vi "Process.vi"(8 "error in (no error)":errorcluster, 11 "Report Generator In":refnum<class "Report Generator.lvclass">) -> (0 "error out":errorcluster, 3 "Report Generator Out":refnum<class "Report Generator.lvclass">)   [LabVIEW 2020, in "Report Generator.lvclass"]
uses:
  Report Generator.lvclass
  C:/Git/astemes-lunit/source/Application Framework/Process Classes/Process/Process.lvclass
  Report Generator.lvclass/Report Generator.ctl
  Report Classes/XML Report/XML Report.lvclass
  Result Collector/Result Collector.lvclass/Result Collector.ctl
  Result Types/Suite Results/Test Suite Result.ctl
  Result Types/Case Result/Test Case Result.ctl
  Result Types/Method Result/Method Result.ctl
  Rewrite Project/Result/Status.ctl
  Result Types/Assertion Result/Assertion Result.ctl
  Result Types/Assertion Result/Public/TypeDefs/Assertion Type.ctl
  Application Framework/Process Classes/Process/Process.lvclass/Process.ctl
  Result Collector/Result Collector.lvclass
  Report Classes/Test Report/Test Report.lvclass/Test Report.ctl
  Report Classes/Test Report/Test Report.lvclass
  Result Types/Suite Results/Public/Read Errors count.vi
  Result Types/Suite Results/Public/Read Test Method Count.vi
  Result Types/Suite Results/Public/Read Test Case count.vi
  Result Types/Suite Results/Public/Read Failed count.vi
  Result Types/Suite Results/Public/Read Execution time.vi
  Result Types/Suite Results/Public/Read Passed count.vi
  Result Types/Suite Results/Public/Read Skipped count.vi
  Application Framework/Process Classes/Process/Public/Accessors/Read Process Name.vi
  Result Types/Suite Results/Private/Count by Status.vi
  Result Types/Case Result/Public/Read Test Method Count.vi
  Result Types/Case Result/Public/Read Status.vi
  Result Types/Case Result/Private/Merge Status.vi
  Result Types/Method Result/Public/Read Status.vi
  <vilib>/Utility/error.llb/Error Cluster From Error Code.vi
  Application Framework/Process Classes/Error Handler/Private/SubVIs/Get Error Queue Name.vi
  Application Framework/Process Classes/Process/Process.lvclass
  Application Framework/Process Classes/Error Handler/Error Handler.lvclass
  Result Types/Case Result/Test Case Result.lvlib
  Result Types/Suite Results/Test Suite Result.lvlib
  Rewrite Project/Result/Result.lvlib
  Result Types/Assertion Result/Assertion Result.lvlib
  Result Types/Method Result/Method Result.lvlib
panel:
  out "Stopped":bool
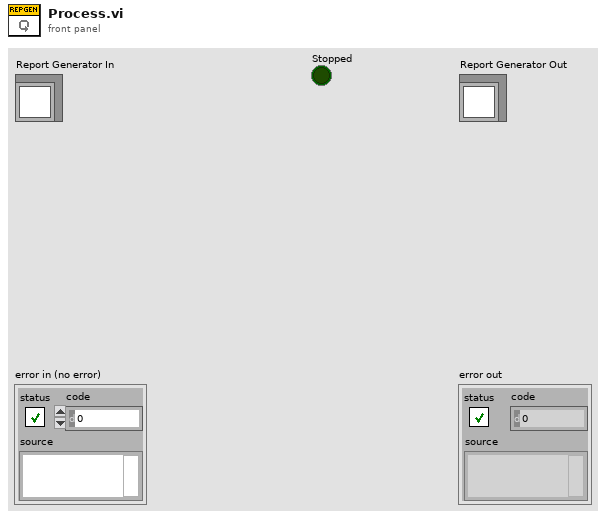
[diagram p1: front panel]
types:
  T1 = typedef "Test Suite Result.lvlib/Test Suite Result.ctl" = cluster{"Test Suite ID":string, "Name":string, "Hostname":string, "Status":T2, "Execution time":dbl, "Start Time":timestamp, "Case Results":T3[]}
  T2 = typedef "Result.lvlib/Status.ctl" = enum16{"Pass", "Fail", "Error", "Skipped", "Setup Error", "Broken", "Teardown Error"}
  T3 = typedef "Test Case Result.lvlib/Test Case Result.ctl" = map{string, T4}
  T4 = typedef "Method Result.lvlib/Method Result.ctl" = cluster{"Test Case":string, "Test Method Name":string, "Status":T2, "Assertion Results":T5[], "Execution time":dbl, "Result String":string}
  T5 = typedef "Assertion Result.lvlib/Assertion Result.ctl" = cluster{"Status":T2, "Message":string, "Description":string, "Assertion Type":T6}
  T6 = typedef "Result.lvlib/Assertion Type.ctl" = enum16{"None", "Pass", "Fail", "Skip", "Pass if Equal", "Fail if Equal", "Pass if Error", "Fail if Error", "Pass if", "Fail if"}
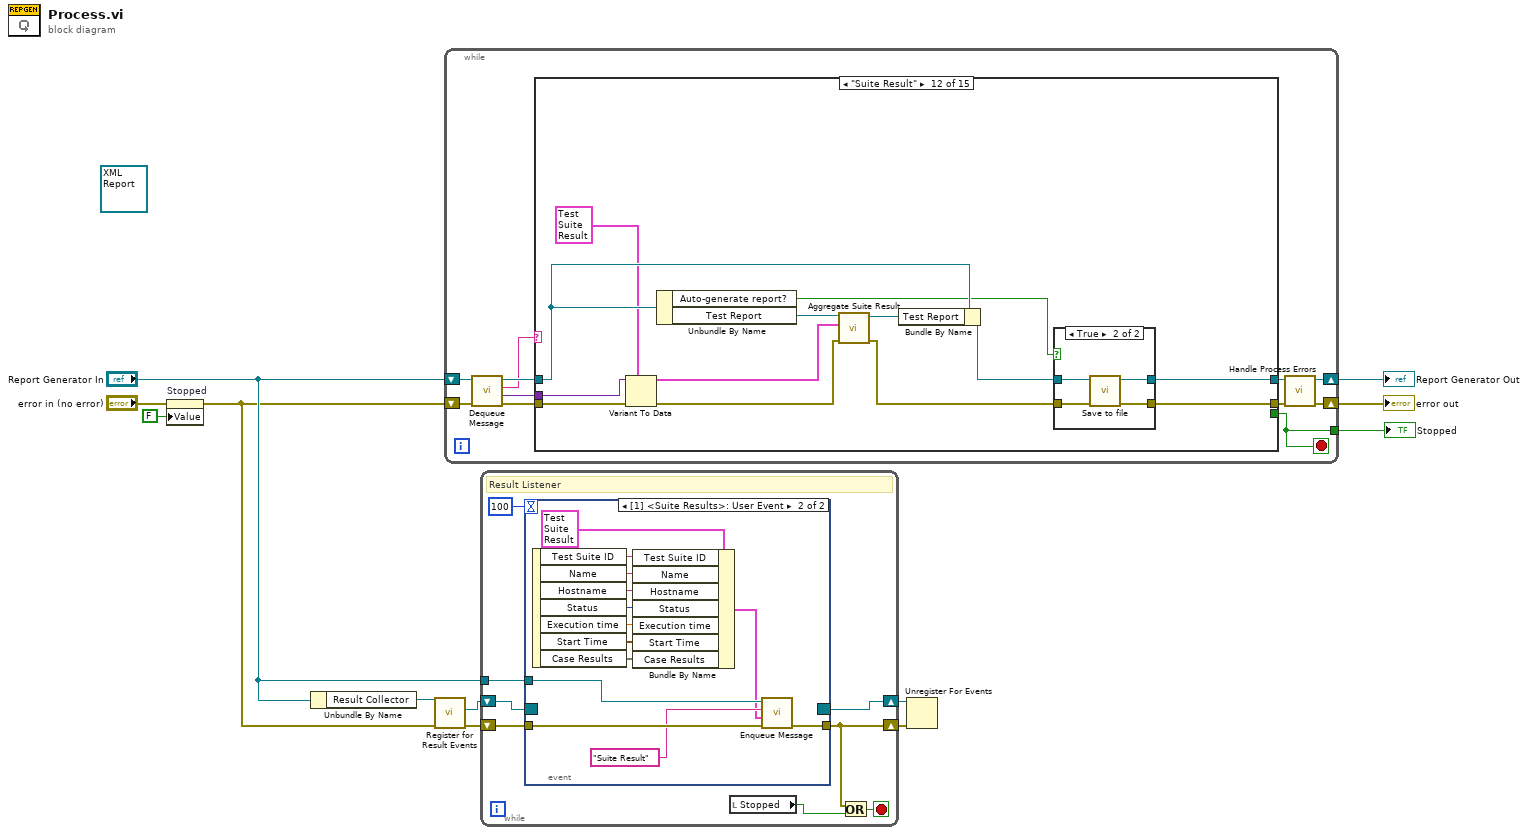
[diagram p0: block diagram]
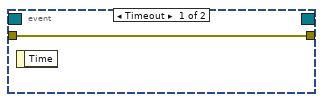
[diagram p2: hidden frame]
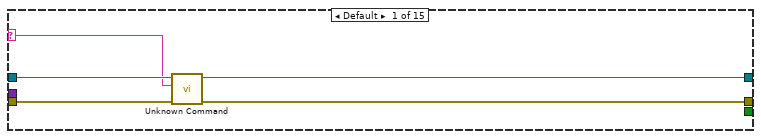
[diagram p3: hidden frame]
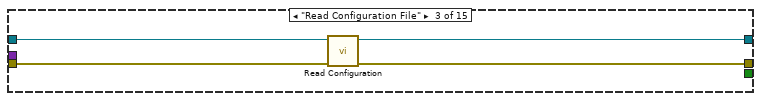
[diagram p5: hidden frame]
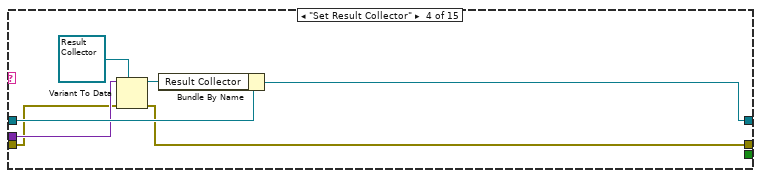
[diagram p6: hidden frame]
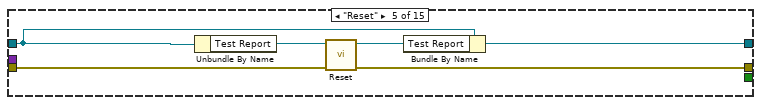
[diagram p7: hidden frame]
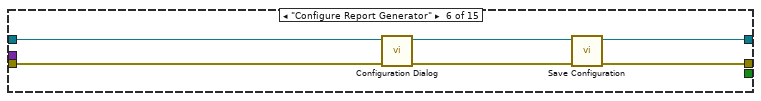
[diagram p8: hidden frame]
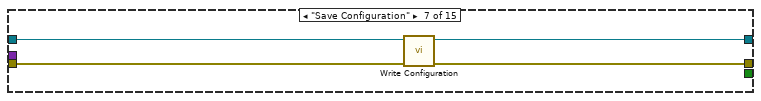
[diagram p9: hidden frame]
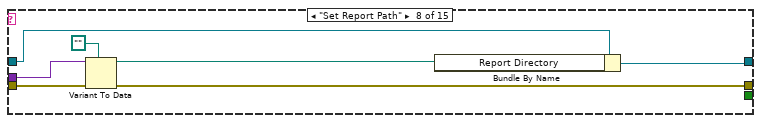
[diagram p10: hidden frame]
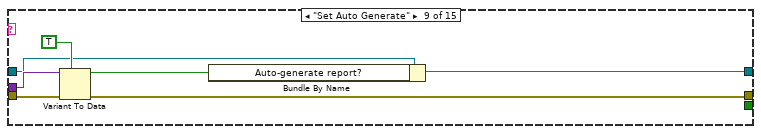
[diagram p11: hidden frame]
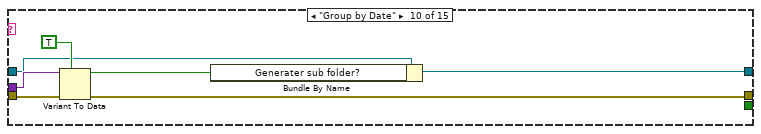
[diagram p12: hidden frame]
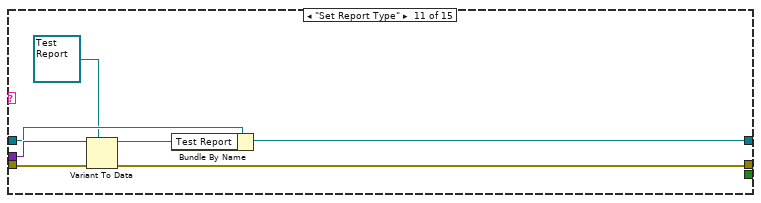
[diagram p13: hidden frame]
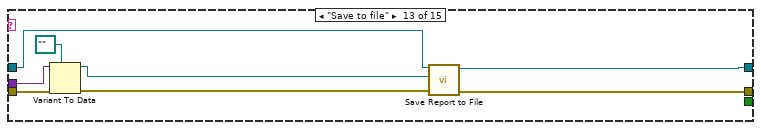
[diagram p15: hidden frame]
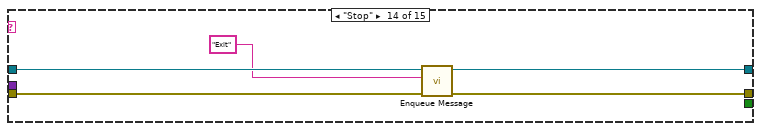
[diagram p16: hidden frame]
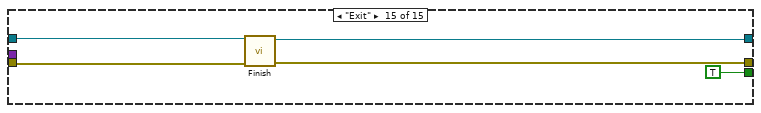
[diagram p17: hidden frame]
diagram:
  (unwired) refnum<class "XML Report.lvclass"> refnum ("XML Report.lvclass")
  n1 = property on="Stopped" class="Bool (strict)"(error in="error in (no error)", "Value"=FALSE ("Stopped")) -> (error out=w1:errorcluster)  [unwired: 1 in, 1 out]
  n2 = Unbundle By Name("Report Generator In") -> ("Result Collector"=w10:refnum<class "Result Collector.lvclass">)
  n3 = call "Register for Result Events.vi"("error in (no error)"=w1, "Result Collector In"=w10) -> ("error out"=w8:errorcluster, "Event Registration Refnum"=w9:refnum<event-registration>)  [unwired: 7 in, 1 out]
  n4 = while {
    shift-right: [w16] -> w12
    shift-left: w1 -> [w22]
    shift-right: [w17] -> w11
    shift-left: "Report Generator In" -> [w23]
    tunnel: [w13] -> w4
    stop <- w13 stop-if-true
    n5 = call "Dequeue Message.vi"("error in (no error)"=w22, "Process In"=w23) -> ("error out"=w21:errorcluster, "Message Data"=w14:variant, "Message"=w18:string, "Process Out"=w19:refnum<class "Report Generator.lvclass">)  [unwired: 6 in]
    n6 = case shown="\"Suite Result\"" w18 {
      selector: w18 -> [w24 _ _ _ _ _ _ _ _ _ _ _ _ _ _]
      tunnel: [w26 w29 w31 w35 w43 w49 w54 w58 w66 w73 w81 w88 w107 w114 w119] -> w15
      tunnel: w21 -> [w25 w29 w32 w39 w44 w52 w55 w64 w71 w78 w85 w96 w112 w116 w121]
      tunnel: [w28 w30 w33 w36 w42 w48 w56 w60 w65 w72 w80 w90 w106 w115 w120] -> w20
      tunnel: w19 -> [w27 w30 w34 w41 w45 w53 w57 w61 w68 w75 w83 w98 w109 w117 w122]
      tunnel: [_ _ _ _ _ _ _ _ _ _ _ _ _ _ TRUE] -> w13
      tunnel: w14 -> [_ _ _ w40 _ _ _ w63 w70 w77 w84 w93 w111 _ _]
      frame Default {
        n7 = call "Unknown Command.vi"("error in (no error)"=w25, "String"=w24, "Process In"=w27) -> ("error out"=w26:errorcluster, "Process Out"=w28:refnum<class "Report Generator.lvclass">)  [unwired: 7 in]
      }
      frame "Init" {
      }
      frame "Read Configuration File" {
        n8 = call-dynamic "Read Configuration.vi"("error in (no error)"=w32, "Report Generator In"=w34) -> ("error out"=w31:errorcluster, "Report Generator Out"=w33:refnum<class "Report Generator.lvclass">)  [unwired: 8 in]
      }
      frame "Set Result Collector" {
        n9 = Variant To Data(error in=w39, type=refnum<class "Result Collector.lvclass"> refnum ("Result Collector"), Variant=w40) -> (data=w37:refnum<class "Result Collector.lvclass">, error out=w35:errorcluster)
        n10 = Bundle By Name(cluster=w41, "Result Collector"=w37) -> (w36:refnum<class "Report Generator.lvclass">)
      }
      frame "Reset" {
        n11 = Unbundle By Name(w45) -> ("Test Report"=w47:refnum<class "Test Report.lvclass">)
        n12 = call "Reset.vi"("error in (no error)"=w44, "Report In"=w47) -> ("error out"=w43:errorcluster, "Report Out"=w46:refnum<class "Test Report.lvclass">)  [unwired: 8 in]
        n13 = Bundle By Name(cluster=w45, "Test Report"=w46) -> (w42:refnum<class "Report Generator.lvclass">)
      }
      frame "Configure Report Generator" {
        n14 = call "Configuration Dialog.vi"("error in (no error)"=w52, "Report Generator In"=w53) -> ("error out"=w50:errorcluster, "Report Generator Out"=w51:refnum<class "Report Generator.lvclass">)  [unwired: 8 in]
        n15 = call "Save Configuration.vi"("error in (no error)"=w50, "Report Generator in"=w51) -> ("error out"=w49:errorcluster, "Report Generator out"=w48:refnum<class "Report Generator.lvclass">)  [unwired: 8 in]
      }
      frame "Save Configuration" {
        n16 = call-dynamic "Write Configuration.vi"("error in (no error)"=w55, "Report Generator In"=w57) -> ("error out"=w54:errorcluster, "Report Generator Out"=w56:refnum<class "Report Generator.lvclass">)  [unwired: 8 in]
      }
      frame "Set Report Path" {
        n17 = Variant To Data(error in=w64, type=path "", Variant=w63) -> (data=w59:path, error out=w58:errorcluster)
        n18 = Bundle By Name(cluster=w61, "Report Directory"=w59) -> (w60:refnum<class "Report Generator.lvclass">)
      }
      frame "Set Auto Generate" {
        n19 = Variant To Data(error in=w71, type=TRUE, Variant=w70) -> (data=w67:bool, error out=w66:errorcluster)
        n20 = Bundle By Name(cluster=w68, "Auto-generate report?"=w67) -> (w65:refnum<class "Report Generator.lvclass">)
      }
      frame "Group by Date" {
        n21 = Variant To Data(error in=w78, type=TRUE, Variant=w77) -> (data=w74:bool, error out=w73:errorcluster)
        n22 = Bundle By Name(cluster=w75, "Generater sub folder?"=w74) -> (w72:refnum<class "Report Generator.lvclass">)
      }
      frame "Set Report Type" {
        n23 = Variant To Data(error in=w85, type=refnum<class "Test Report.lvclass"> refnum ("Test Report.lvclass"), Variant=w84) -> (data=w82:refnum<class "Test Report.lvclass">, error out=w81:errorcluster)
        n24 = Bundle By Name(cluster=w83, "Test Report"=w82) -> (w80:refnum<class "Report Generator.lvclass">)
      }
      frame "Suite Result" {
        n25 = Variant To Data(error in=w96, type=T1 {"Test Suite ID"="", "Name"="", "Hostname"="", "Status"=enum."Pass", "Execution time"=0.0, "Start Time"=timestamp(0 s since 1904-01-01), "Case Results"=[]} ("Cluster of class private data"), Variant=w93) -> (data=w92:T1, error out=w94:errorcluster)
        n26 = Unbundle By Name(w98) -> ("Auto-generate report?"=w87:bool, "Test Report"=w97:refnum<class "Test Report.lvclass">)
        n27 = call "Aggregate Suite Result.vi"("error in (no error)"=w94, "Test Suite Result"=w92, "Report In"=w97) -> ("error out"=w89:errorcluster, "Report Out"=w95:refnum<class "Test Report.lvclass">)  [unwired: 7 in]
        n28 = Bundle By Name(cluster=w98, "Test Report"=w95) -> (w91:refnum<class "Report Generator.lvclass">)
        n29 = case shown="True" w87 {
          tunnel: w91 -> [w100 w104]
          tunnel: [w100 w103] -> w90
          tunnel: w89 -> [w99 w102]
          tunnel: [w99 w101] -> w88
          frame False {
          }
          frame True {
            n30 = call "Save to file.vi"("error in (no error)"=w102, "Report Generator In"=w104) -> ("error out"=w101:errorcluster, "Report Generator Out"=w103:refnum<class "Report Generator.lvclass">)  [unwired: 8 in]
          }
        }
      }
      frame "Save to file" {
        n31 = Variant To Data(error in=w112, type=path "", Variant=w111) -> (data=w105:path, error out=w108:errorcluster)
        n32 = call "Save Report to File.vi"("error in (no error)"=w108, "Report Directory"=w105, "Report Generator in"=w109) -> ("error out"=w107:errorcluster, "Report Generator out"=w106:refnum<class "Report Generator.lvclass">)  [unwired: 7 in]
      }
      frame "Stop" {
        n33 = call "Enqueue Message.vi"("error in (no error)"=w116, "Message"="Exit", "Process In"=w117) -> ("error out"=w114:errorcluster, "Process Out"=w115:refnum<class "Report Generator.lvclass">)  [unwired: 7 in]
      }
      frame "Exit" {
        n34 = call "Finish.vi"("error in (no error)"=w121, "Process In"=w122) -> ("error out"=w119:errorcluster, "Process Out"=w120:refnum<class "Report Generator.lvclass">)  [unwired: 8 in]
      }
    }
    n35 = call "Handle Process Errors.vi"("error in (no error)"=w15, "Process In"=w20) -> ("error out"=w16:errorcluster, "Process Out"=w17:refnum<class "Report Generator.lvclass">)  [unwired: 8 in]
  }
  "error out" <- w12
  "Report Generator Out" <- w11
  "Stopped" <- w4
  n36 = while {
    tunnel: "Report Generator In" -> [w128]
    shift-right: [w127] -> w6
    shift-left: w9 -> [w130]
    shift-right: [w125] -> w5
    shift-left: w8 -> [w129]
    stop <- w124 stop-if-true
    # "Result Listener"
    n37 = event shown="[1] <Suite Results>: User Event" {
      selector: w130 -> [_ _]
      dyn-events: [_ _] -> w127
      timeout: 100 -> [_ _]
      tunnel: w129 -> [w131 w144]
      tunnel: w128 -> [_ w143]
      tunnel: [w131 w141] -> w125
      event Timeout {
        n38 = event-data() -> ()  [unwired: 1 in, 1 out]
      }
      event User Event {
        n39 = event-data() -> ("Test Suite ID"=w139:string, "Name"=w138:string, "Hostname"=w137:string, "Status"=w136:T2, "Execution time"=w135:dbl, "Start Time"=w134:timestamp, "Case Results"=w133:T3[])  [unwired: 1 in]
        n40 = Bundle By Name(cluster=T1 {"Test Suite ID"="", "Name"="", "Hostname"="", "Status"=enum."Pass", "Execution time"=0.0, "Start Time"=timestamp(0 s since 1904-01-01), "Case Results"=[]} ("Cluster of class private data"), "Test Suite ID"=w139, "Name"=w138, "Hostname"=w137, "Status"=w136, "Execution time"=w135, "Start Time"=w134, "Case Results"=w133) -> (w132:T1)
        n41 = call "Enqueue Message.vi"("error in (no error)"=w144, "Message Data"=w132, "Message"="Suite Result", "Process In"=w143) -> ("error out"=w141:errorcluster)  [unwired: 6 in, 1 out]
      }
    }
    n42 = local read "Stopped"() -> (w123:bool)
    n43 = Or(x=w125, y=w123) -> (x .or. y?=w124:bool)
  }
  n44 = Unregister For Events(event registration refnum=w6, error in=w5) -> ()  [unwired: 1 out]
